vi "decodeStatus.vi"(8 "error in (no error)":errorcluster, 11 "Data":i16[](array[numeric])) -> (0 "error out":errorcluster, 3 "String":string)   [LabVIEW 2017]
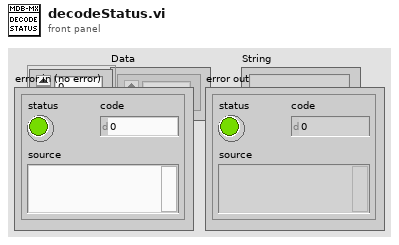
[diagram p1: front panel]
types:
  T1 = cluster{"Stop":bool, "Forward Running":bool, "Reverse Running":bool, "Fault(Trip)":bool, "Acceleration":bool, "Deceleration":bool, "Speed Arrived":bool, "DC Braking":bool, "Stopping":bool, "Brake Open":bool, "Forward run Command":bool, "Reverse run Command":bool}
  T2 = cluster{"Current":dbl, "Freq":dbl, "Voltage":dbl, "DC Link":dbl, "Power":dbl, "Flags":cluster{"Stop":bool, "Forward Running":bool, "Reverse Running":bool, "Fault(Trip)":bool, "Acceleration":bool, "Deceleration":bool, "Speed Arrived":bool, "DC Braking":bool, "Stopping":bool, "Brake Open":bool, "Forward run Command":bool, "Reverse run Command":bool}}
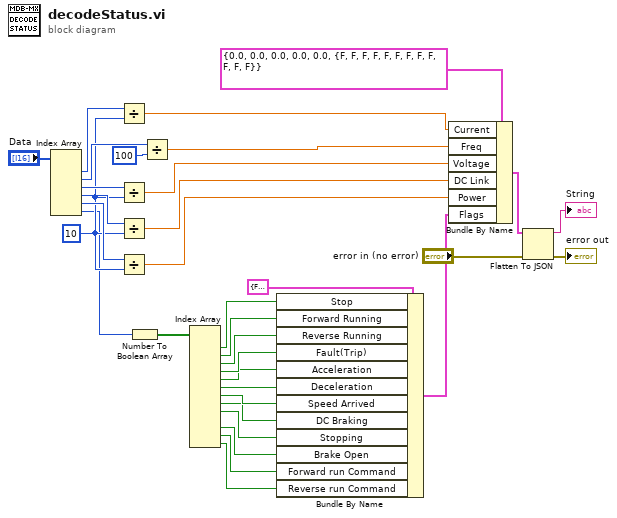
[diagram p0: block diagram]
diagram:
  w28 = i16 10 ("y")
  n1 = Index Array(array="Data") -> (element #1=w33:i16, element #2=w32:i16, element #3=w31:i16, element #4=w30:i16, element #5=w29:i16, element #6=w18:i16)  [unwired: 6 in]
  n2 = Divide(x=w33, y=w28) -> (x/y=w25:dbl)
  n3 = Divide(x=w31, y=w28) -> (x/y=w23:dbl)
  n4 = Divide(x=w30, y=w28) -> (x/y=w22:dbl)
  n5 = Divide(x=w29, y=w28) -> (x/y=w21:dbl)
  n6 = Number To Boolean Array(number=w18) -> (Boolean array=w17:bool[])
  n7 = Divide(x=w32, y=i16 100) -> (x/y=w24:dbl)
  n8 = Index Array(array=w17) -> (element #1=w16:bool, element #2=w15:bool, element #3=w14:bool, element #4=w13:bool, element #5=w12:bool, element #6=w11:bool, element #7=w10:bool, element #8=w9:bool, element #9=w8:bool, element #11=w7:bool, element #12=w6:bool, element #13=w5:bool)  [unwired: 13 in, 1 out]
  n9 = Bundle By Name(cluster=T1 {"Stop"=FALSE, "Forward Running"=FALSE, "Reverse Running"=FALSE, "Fault(Trip)"=FALSE, "Acceleration"=FALSE, "Deceleration"=FALSE, "Speed Arrived"=FALSE, "DC Braking"=FALSE, "Stopping"=FALSE, "Brake Open"=FALSE, "Forward run Command"=FALSE, "Reverse run Command"=FALSE}, "Stop"=w16, "Forward Running"=w15, "Reverse Running"=w14, "Fault(Trip)"=w13, "Acceleration"=w12, "Deceleration"=w11, "Speed Arrived"=w10, "DC Braking"=w9, "Stopping"=w8, "Brake Open"=w7, "Forward run Command"=w6, "Reverse run Command"=w5) -> (w19:T1)
  n10 = Bundle By Name(cluster=T2 {"Current"=0.0, "Freq"=0.0, "Voltage"=0.0, "DC Link"=0.0, "Power"=0.0, "Flags"={"Stop"=FALSE, "Forward Running"=FALSE, "Reverse Running"=FALSE, "Fault(Trip)"=FALSE, "Acceleration"=FALSE, "Deceleration"=FALSE, "Speed Arrived"=FALSE, "DC Braking"=FALSE, "Stopping"=FALSE, "Brake Open"=FALSE, "Forward run Command"=FALSE, "Reverse run Command"=FALSE}}, "Current"=w25, "Freq"=w24, "Voltage"=w23, "DC Link"=w22, "Power"=w21, "Flags"=w19) -> (w4:T2)
  n11 = Flatten To JSON(anything=w4, error in (no error)="error in (no error)") -> (JSON string=→"String":string, 11:→"error out":errorcluster)  [unwired: 1 in]
